vi "简易流程启动.vi"(8 "Error in":errorcluster caption="Error in (no error)", 9 "简易流程":u16(ring), 10 "参数Id":u16, 11 "MB session in":refnum<class "MB_Master.lvclass">) -> (0 "error out":errorcluster, 3 "MB session out":refnum<class "MB_Master.lvclass">)   [LabVIEW 2016, in "斯坦道总磷总氮.lvlib"]
uses:
  <vilib>/Plasmionique/MB Master/MB_Master/MB_Master.lvclass
  <vilib>/Plasmionique/MB Master/MB Master.lvlib
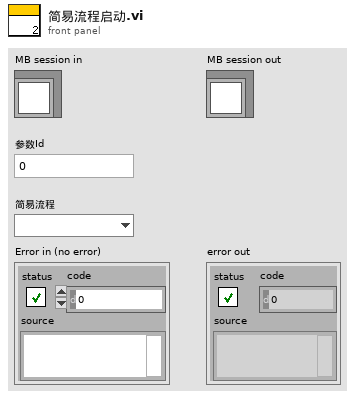
[diagram p1: front panel]
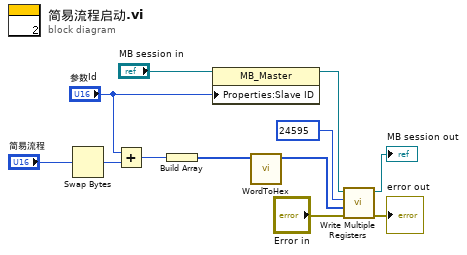
[diagram p0: block diagram]
diagram:
  n1 = Swap Bytes(anything="简易流程") -> (byte swapped=w6:u16)
  n2 = Add(x="参数Id", y=w6) -> (x+y=w5:u16)
  n3 = Build Array(w5) -> (w4:u16[])
  n4 = property class="MB_Master"(reference="MB session in", "Properties:Slave ID"="参数Id") -> (reference out=w2:refnum<class "MB_Master.lvclass">)  [unwired: 1 in, 1 out]
  n5 = call "WordToHex.vi"("WORD"=w4) -> ("数组"=w8:u16[])  [unwired: 10 in]
  n6 = call <vilib>:"Write Multiple Registers.vi"("error in (no error)"="Error in", "values"=w8, "starting address"=u16 24595, "MB session in"=w2) -> ("error out"=→"error out":errorcluster, "MB session out"=→"MB session out":refnum<class "MB_Master.lvclass">)  [unwired: 6 in]
